vi "Scenario Delete.vi"(8 "error in (no error)":errorcluster, 10 "ixScenario (0)":i32, 11 "Connection Refnum":T1) -> (0 "error out":errorcluster, 3 "Connection Refnum":T1)   [LabVIEW 2011]
uses:
  Summitek EXT/ODBC/SQL Controls/Connection Refnum.ctl
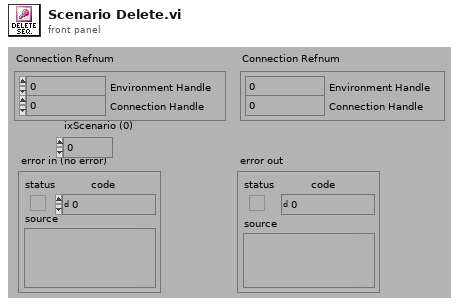
[diagram p1: front panel]
types:
  T1 = typedef "Connection Refnum.ctl" = cluster{"Environment Handle":i32, "Connection Handle":i32}
  T2 = typedef "Statement Refnum.ctl" = cluster{"Statement Handle":i32, "Parameter Number":u16}
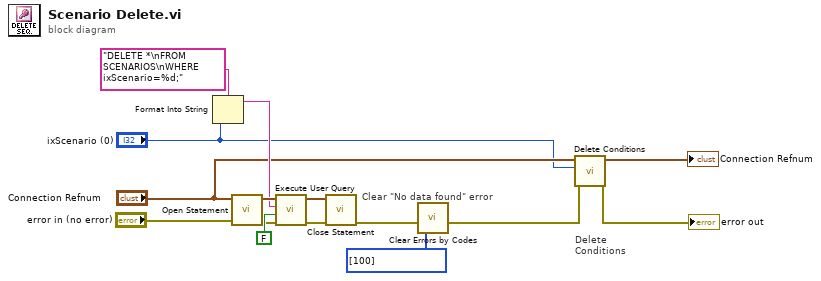
[diagram p0: block diagram]
diagram:
  # "Clear \"No data found\" error"
  # "Delete\nConditions"
  n1 = Format Into String(format string="DELETE *\nFROM SCENARIOS\nWHERE ixScenario=%d;" ("User Query"), "ixScenario (0)") -> (resulting string=w9:string)  [unwired: 2 in, 1 out]
  n2 = call "Open Statement.vi"("error in (no error)"="error in (no error)", "Connection Refnum"="Connection Refnum") -> ("error out"=w11:errorcluster, "Statement Refnum"=w10:T2)  [unwired: 4 out]
  n3 = call "Execute User Query.vi"("error in (no error)"=w11, "Return Data? (f)"=FALSE, "User Query"=w9, "Statement Refnum"=w10) -> ("error out"=w13:errorcluster, "Statement Refnum"=w14:T2)  [unwired: 2 out]
  n4 = call "Close Statement.vi"("error in (no error)"=w13, "Statement Refnum"=w14) -> ("error out"=w7:errorcluster)  [unwired: 5 out]
  n5 = call "Clear Errors by Codes.vi"("Error Codes\nto Clear (Empty)"=i32[] [100] ("Error Codes\nto Clear (Empty)"), "error in (no error)"=w7) -> ("error out"=w4:errorcluster)  [unwired: 5 out]
  n6 = call "Delete Conditions.vi"("error in (no error)"=w4, "ixScenario (0)"="ixScenario (0)", "Connection Refnum"="Connection Refnum") -> ("error out"=→"error out":errorcluster, "Connection Refnum"=→"Connection Refnum":T1)  [unwired: 7 out]
